vi "Add Polynomials (DBL).vi"(8 "threshold type":T1 items=["Absolute Value", "Relative Value"], 9 "threshold":dbl, 10 "Q(x)":dbl[](array[numeric]) format="%#.6g", 11 "P(x)":dbl[](array[numeric]) format="%#.6g") -> (0 "error":i32, 3 "P(x)+Q(x)":dbl[](array[numeric]) format="%#.6g")   [LabVIEW 2010, in "NI_AALPro.lvlib"]
doc: "Adds two polynomials <B>P(x)</B> and <B>Q(x)</B>. The data types you wire to the <B>P(x)</B> and <B>Q(x)</B> inputs determine the polymorphic instance to use."
uses:
  NI_AALPro.lvlib
  Remove Zero Threshold Type.ctl
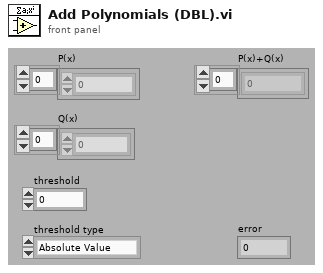
[diagram p1: front panel]
types:
  T1 = typedef "NI_AALPro.lvlib/Remove Zero Threshold Type.ctl" = u16
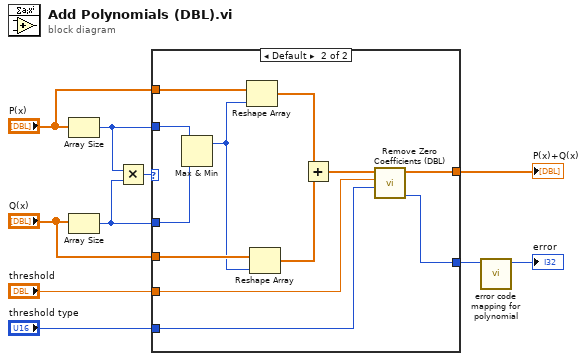
[diagram p0: block diagram]
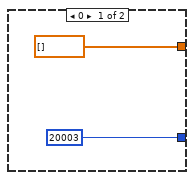
[diagram p2: hidden frame]
diagram:
  n1 = Array Size(array="P(x)") -> (size(s)=w6:i32)
  n2 = Array Size(array="Q(x)") -> (size(s)=w5:i32)
  n3 = Multiply(x=w6, y=w5) -> (x*y=w7:i32)
  n4 = case shown="Default" w7 {
    tunnel: w6 -> [_ w24]
    tunnel: w5 -> [_ w23]
    tunnel: "P(x)" -> [_ w19]
    tunnel: "Q(x)" -> [_ w17]
    tunnel: [dbl[] [] w21] -> w8
    tunnel: [20003 ("empty array") w20] -> w4
    tunnel: "threshold" -> [_ w14]
    tunnel: "threshold type" -> [_ w13]
    frame 0 {
    }
    frame Default {
      n5 = Max & Min(x=w24, y=w23) -> (max(x,y)=w16:i32)  [unwired: 1 out]
      n6 = Reshape Array(w19, w16) -> (w18:dbl[])
      n7 = Reshape Array(w17, w16) -> (w15:dbl[])
      n8 = Add(x=w18, y=w15) -> (x+y=w22:dbl[])
      n9 = call "Remove Zero Coefficients (DBL).vi"("threshold type"=w13, "threshold"=w14, "P(x) In"=w22) -> ("error"=w20:i32, "P(x) Out"=w21:dbl[])  [unwired: 6 in, 1 out]
    }
  }
  "P(x)+Q(x)" <- w8
  n10 = call "error code mapping for polynomial.vi"("error in"=w4) -> ("error out"=→"error":i32)  [unwired: 10 in]
